vi "FTW-HTTPClient-CloseConnection.vi"(0 "HTTP Client":refnum<class "FTW-HTTPClient.lvclass">, 11 "error in":errorcluster) -> (15 "error out":errorcluster)   [LabVIEW 2012, in "FTW-HTTPClient.lvclass"]
uses:
  FTW-HTTPClient.lvclass
  FTW-HTTPClient.lvclass/FTW-HTTPClient.ctl
panel:
  # "Inputs"
  # "Outputs"
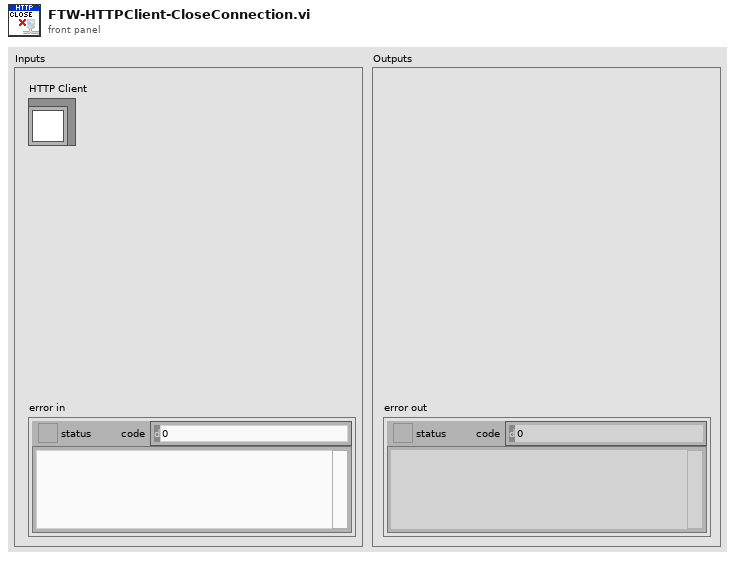
[diagram p1: front panel]
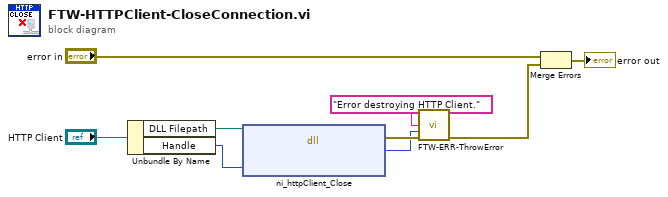
[diagram p0: block diagram]
diagram:
  n1 = Unbundle By Name("HTTP Client") -> ("DLL Filepath"=w6:path, "Handle"=w5:u32)
  n2 = dll-call lib="?" fn="ni_httpClient_Close"(path in=w6, "Handle"=w5) -> (error out=w4:errorcluster, "Return"=w3:i32)  [unwired: 3 in, 1 out]
  n3 = call "FTW-ERR-ThrowError.vi"("Error Message"="Error destroying HTTP Client.", "Error Code"=w3, "error in"=w4) -> ("error out"=w1:errorcluster)  [unwired: 12 in]
  n4 = Merge Errors("error in", w1) -> (→"error out":errorcluster)
